vi "component_changes.vi"(1 "Component Type":T2, 2 "Old Component List":string[](array[string]), 3 "New Component List":string[](array[string])) -> (0 "Component Changes":T1(array[cluster]))   [LabVIEW 2015]
uses:
  ComponentType.ctl
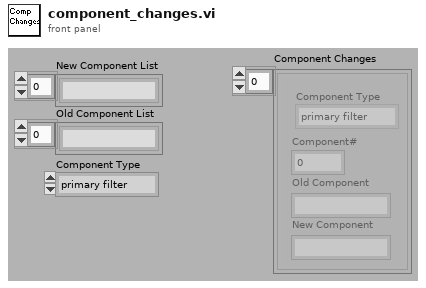
[diagram p1: front panel]
types:
  T1 = cluster{"Component Type":enum16{"primary filter", "secondary filter", "grating", "slit/mask"}, "Component#":i32, "Old Component":string, "New Component":string}[]
  T2 = typedef "ComponentType.ctl" = enum16{"primary filter", "secondary filter", "grating", "slit/mask"}
  T3 = cluster{"Component Type":T2, i32, "String":string, "String":string}
  T4 = cluster{"Component Type":T2, "Component#":i32, "String":string, "String":string}[]
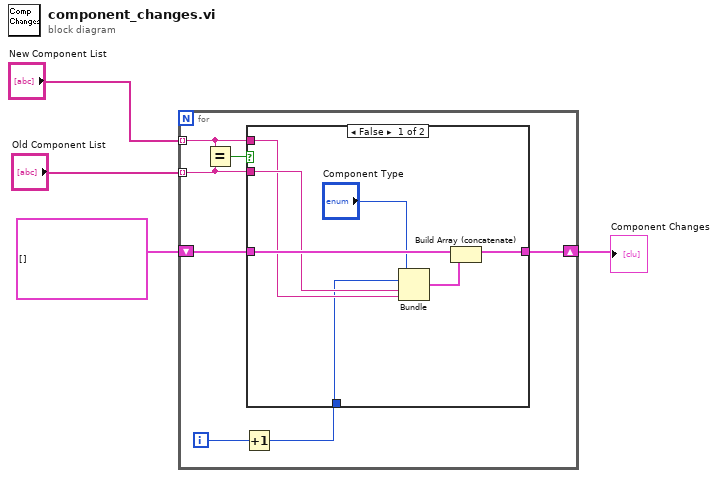
[diagram p0: block diagram]
diagram:
  n1 = for {
    shift-right: [w10] -> w2
    shift-left: T1 [] ("Component Changes") -> [w11]
    tunnel: "Old Component List" -> [w7] mode=indexing
    tunnel: "New Component List" -> [w8] mode=indexing
    i -> [w6]
    n2 = Equal?(x=w8, y=w7) -> (x = y?=w9:bool)
    n3 = Increment(x=w6) -> (x+1=w5:i32)
    n4 = case shown="False" w9 {
      tunnel: w11 -> [w18 w19]
      tunnel: [w17 w19] -> w10
      tunnel: w8 -> [w15 _]
      tunnel: w7 -> [w16 _]
      tunnel: w5 -> [w14 _]
      frame False {
        n5 = Bundle("Component Type"="Component Type", w14, "String"=w16, "String"=w15) -> (w12:T3)  [unwired: 1 in]
        n6 = Build Array (concatenate)(w18, w12) -> (w17:T4)
      }
      frame True {
      }
    }
  }
  "Component Changes" <- w2
